vi "CC Install Config File.vi"() -> (2 "Hardware Config out":T1, 3 "new path":path)   [LabVIEW 2022 SP3]
uses:
  typedefs/CC cluster Hardware Config.ctl
  typedefs/CC cluster Device Index.ctl
panel:
  in  "OK Button":bool
  in  "Select Install Type":enum16{"Simulation", "Full Standard Hardware"}(ring)
  # "RIMAS Camera Control"
  # "No configuration file found. Select configuration from list below. Simulation mode will simulate all subsystem hardware. Full Standard Hardware attempts to communicate with all subsystems.\n\nHardware selections can be changed at anytime using the Settings-->Select Hardware menu option."
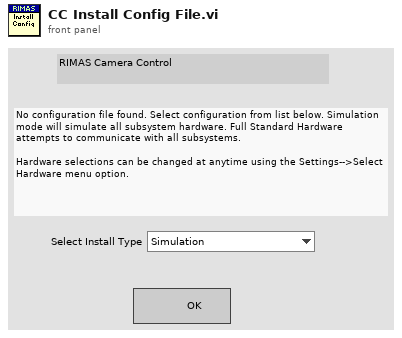
[diagram p1: front panel]
types:
  T1 = typedef "CC cluster Hardware Config.ctl" = cluster{"Installed Hardware":T2[]}
  T2 = typedef "CC cluster Device Index.ctl" = cluster{"Device Type Name":string, "Curr Device Name":string, "All Instances":string[]}
  T3 = enum32{"Invalid", "Standard", "Closed", "Hidden", "Minimized", "Maximized"}
  T4 = enum32{"invalid app kind", "Development System", "Run Time System", "Student Edition", "Embedded LabVIEW", "Evaluation", "Custom"}
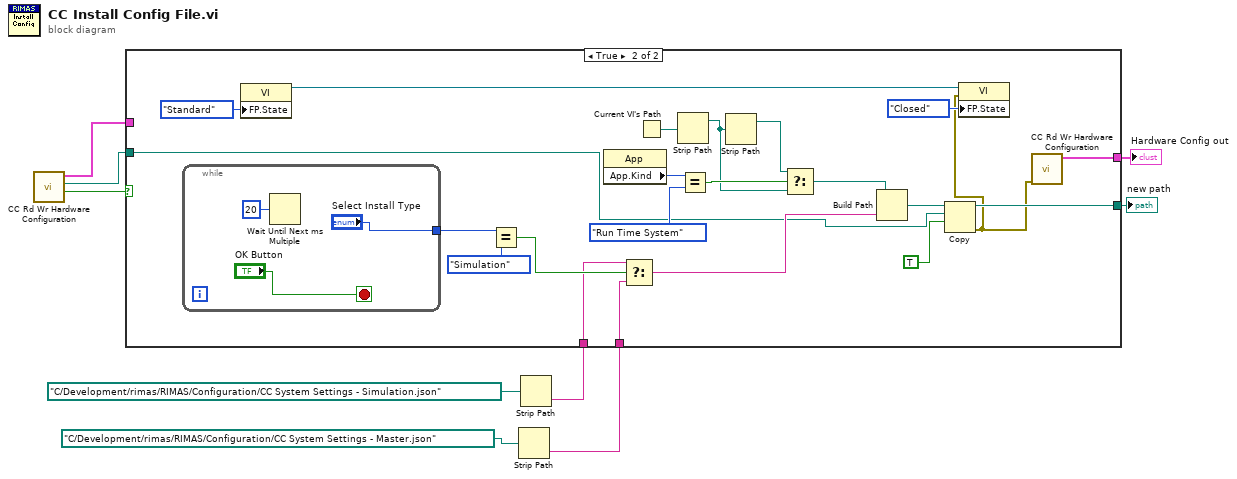
[diagram p0: block diagram]
diagram:
  n1 = call "CC Rd Wr Hardware Configuration.vi"() -> ("New File?"=w9:bool, "File"=w7:path, "Hardware Config out"=w8:T1)  [unwired: 8 in, 1 out]
  n2 = Strip Path(path=path "C:/Development/rimas/RIMAS/Configuration/CC System Settings - Master.json" ("Path")) -> (name=w3:string)  [unwired: 1 out]
  n3 = Strip Path(path=path "C:/Development/rimas/RIMAS/Configuration/CC System Settings - Simulation.json" ("Path")) -> (name=w4:string)  [unwired: 1 out]
  n4 = case shown="True" w9 {
    tunnel: w8 -> [w10 _]
    tunnel: w7 -> [w11 w18]
    tunnel: w4 -> [_ w22]
    tunnel: w3 -> [_ w21]
    tunnel: [w11 w14] -> w2
    tunnel: [w10 w12] -> w1
    frame False {
    }
    frame True {
      n5 = while {
        tunnel: ["Select Install Type"] -> w30
        stop <- "OK Button" stop-if-true
        n6 = Wait Until Next ms Multiple(millisecond multiple=u32 20) -> ()  [unwired: 1 out]
      }
      n7 = property class="VI"("FP.State"=T3."Standard" ("Front Panel Window:State")) -> (reference out=w16:refnum<vi>)  [unwired: 2 in, 1 out]
      n8 = Equal?(x=w30, y=enum16{"Simulation", "Full Standard Hardware"}."Simulation") -> (x = y?=w23:bool)
      n9 = property class="App"() -> ("App.Kind"=w32:T4)  [unwired: 2 in, 2 out]
      n10 = Select(t=w22, s=w23, f=w21) -> (s? t:f=w20:string)
      n11 = Current VI's Path() -> (path=w28:path)
      n12 = Strip Path(path=w28) -> (stripped path=w26:path)  [unwired: 1 out]
      n13 = Equal?(x=w32, y=T4."Run Time System") -> (x = y?=w27:bool)
      n14 = Strip Path(path=w26) -> (stripped path=w25:path)  [unwired: 1 out]
      n15 = Select(t=w25, s=w27, f=w26) -> (s? t:f=w24:path)
      n16 = Build Path(base path=w24, name or relative path=w20) -> (appended path=w19:path)
      n17 = Copy(9:TRUE ("overwrite (F)"), 10:w18, 11:w19) -> (0:w13:errorcluster, 3:w14:path)  [unwired: 2 in, 1 out]
      n18 = property class="VI"(reference=w16, error in=w13, "FP.State"=T3."Closed" ("Front Panel Window:State")) -> ()  [unwired: 2 out]
      n19 = call "CC Rd Wr Hardware Configuration.vi"("error in (no error)"=w13) -> ("Hardware Config out"=w12:T1)  [unwired: 7 in, 3 out]
    }
  }
  "new path" <- w2
  "Hardware Config out" <- w1
